vi "Initialize.vi"(7 "Serial Configuration":T1={"Baud Rate"=9600, "Parity"=0, "Data Bits"=8, "Stop Bits"=10} {"Stop Bits" items=["1.0"=10]; "Data Bits" items=["8"=8]; "Parity" items=["None", "Odd", "Even"]; "Baud Rate" items=["4800"=4800, "9600"=9600, "19200"=19200, "38400"=38400]}, 8 "error in (no error)":errorcluster, 10 "Communication Address (0)":u8 max=254 format="%x", 11 "VISA resource name":refnum<visa-resource-name>) -> (0 "error out":errorcluster, 3 "VISA resource name out":refnum<visa-resource-name>)   [LabVIEW 2015, in "BK Precision 178XB Series.lvlib"]
doc: "Establishes communication with the instrument and optionally performs an instrument identification query and/or an instrument reset. It also places the instrument in a default state needed for other instrument driver operations. Therefore, call this VI before calling other instrument driver VIs for this instrument. Generally, you need to call the <B>Initialize VI</B> only once at the beginning of an application."
uses:
  <instrlib>/BK Precision 178XB Series/BK Precision 178XB Series.lvlib
panel:
  # "(c) 2009 B&K PRECISION CORPORATION.  ALL RIGHTS RESERVED."
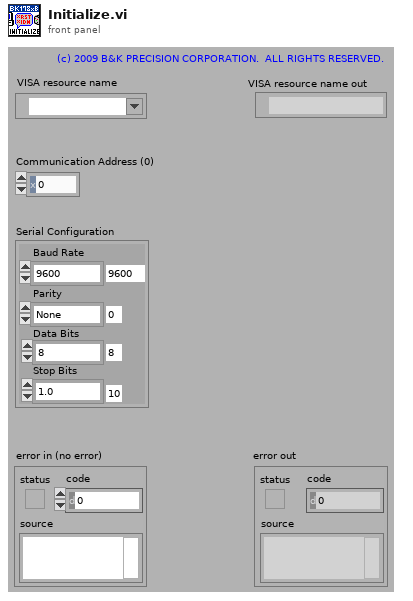
[diagram p1: front panel]
types:
  T1 = cluster{"Baud Rate":u32, "Parity":u16, "Data Bits":u16, "Stop Bits":u16}
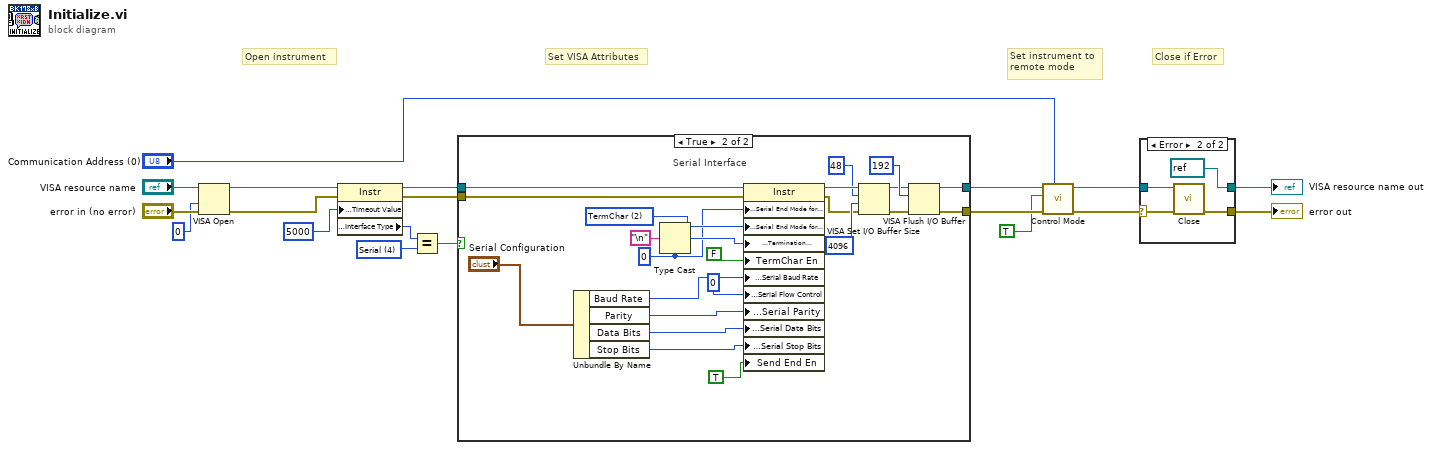
[diagram p0: block diagram]
diagram:
  w12 = u16 4 items=["GPIB"=1, "VXI"=2, "GPIB-VXI"=3, "Serial"=4, "PXI"=5, "TCPIP"=6, "USB"=7] ("Interface Information:Interface Type")
  # "Set instrument to\nremote mode"
  # "Set VISA Attributes"
  # "Close if Error"
  # "Open instrument"
  n1 = VISA Open(access mode=u32 0, error in (no error)="error in (no error)", VISA resource name="VISA resource name") -> (VISA resource name=w8:refnum<visa-resource-name>, error out=w7:errorcluster)  [unwired: 2 in]
  n2 = property class="Instr"(reference=w8, error in=w7, "General Settings:Timeout Value"=u32 5000) -> (reference out=w15:refnum<visa-resource-name>, error out=w14:errorcluster, "Interface Information:Interface Type"=w17:u16)
  n3 = Equal?(x=w17, y=w12) -> (x = y?=w13:bool)
  n4 = case shown="True" w13 {
    tunnel: [w20 w25] -> w5
    tunnel: [w21 w26] -> w6
    tunnel: w15 -> [w20 w43]
    tunnel: w14 -> [w21 w44]
    frame False {
      # "GPIB, TCP/IP, and USB Interface"
    }
    frame True {
      w23 = u8 0
      w40 = u16 2 items=["None", "LastBit", "TermChar"] ("Serial Settings:Serial End Mode for Reads")
      # "Serial Interface"
      n5 = Unbundle By Name("Serial Configuration") -> ("Baud Rate"=w38:u32, "Parity"=w36:u16, "Data Bits"=w37:u16, "Stop Bits"=w34:u16)
      n6 = Type Cast(type=w23, x="\n" ("Line Feed Constant")) -> (*(type *) &x=w39:u8)
      n7 = property class="Instr"(reference=w43, error in=w44, "Serial Settings:Serial End Mode for Reads"=w23, "Serial Settings:Serial End Mode for Writes"=w40, "Message Based Settings:Termination Character"=w39, "TermChar En"=FALSE, "Serial Settings:Serial Baud Rate"=w38, "Serial Settings:Serial Flow Control"=u8 0, "Serial Settings:Serial Parity"=w36, "Serial Settings:Serial Data Bits"=w37, "Serial Settings:Serial Stop Bits"=w34, "Send End En"=TRUE) -> (reference out=w30:refnum<visa-resource-name>, error out=w31:errorcluster)
      n8 = VISA Set I/O Buffer Size(VISA resource name=w30, mask (16)=u32 48 ("size (0)"), size (4096)=u32 4096 ("size (0)"), error in (no error)=w31) -> (VISA resource name out=w28:refnum<visa-resource-name>, error out=w27:errorcluster)
      n9 = VISA Flush I/O Buffer(VISA resource name=w28, mask (16)=u16 192, error in (no error)=w27) -> (VISA resource name out=w25:refnum<visa-resource-name>, error out=w26:errorcluster)
    }
  }
  n10 = call <instrlib>:"Control Mode.vi"("Communication Address (0)"="Communication Address (0)", "error in (no error)"=w6, "Enable Remote Mode (F: Off)"=TRUE, "VISA resource name"=w5) -> ("error out"=w1:errorcluster, "VISA resource name out"=w2:refnum<visa-resource-name>)  [unwired: 6 in]
  n11 = case shown="Error" w1 {
    selector: w1 -> [w45 w48]
    tunnel: w2 -> [w46 w49]
    tunnel: [w46 refnum<visa-resource-name> refnum ("VISA resource name out")] -> w10
    tunnel: [w45 w50] -> w9
    frame No Error {
    }
    frame Error {
      n12 = call "Close.vi"("error in (no error)"=w48, "VISA resource name"=w49) -> ("error out"=w50:errorcluster)  [unwired: 9 in]
    }
  }
  "VISA resource name out" <- w10
  "error out" <- w9
